vi "CSV2_write portion (SubVI).vi"(5 "format (%.3f)":string="%.3f", 6 "delimiter (\\t)":string="\t", 7 "2D data":dbl[][](array[numeric]) format="%0.2f", 8 "error in (no error)":errorcluster, 9 "transpose? (no:F)":bool, 10 "1D data":dbl[](array[numeric]) format="%0.2f", 11 "File Refnum in":refnum<file>) -> (0 "error out":errorcluster, 3 "File Refnum out":refnum<file>)   [LabVIEW 2012]
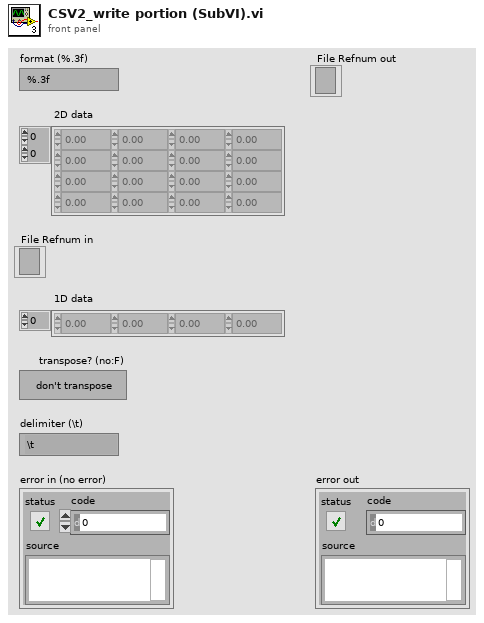
[diagram p1: front panel]
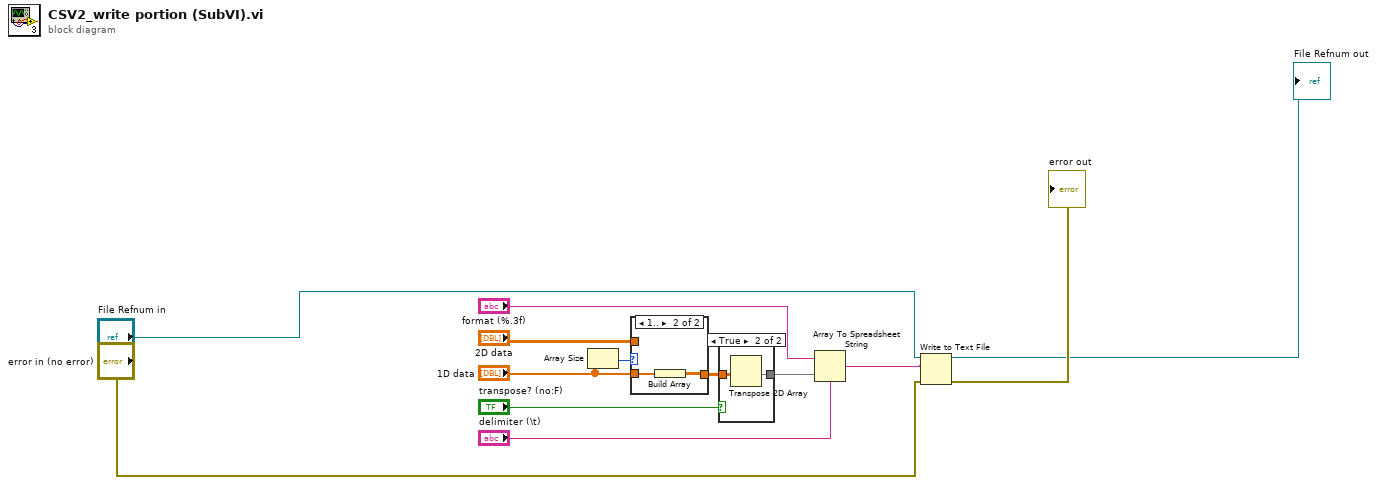
[diagram p0: block diagram]
diagram:
  n1 = Array Size(array="1D data") -> (size(s)=w8:i32)
  n2 = case shown="1.." w8 {
    tunnel: "1D data" -> [_ w16]
    tunnel: [w14 w15] -> w4
    tunnel: "2D data" -> [w14 _]
    frame ..0 {
      # "1D array is empty"
    }
    frame 1.. {
      n3 = Build Array(w16) -> (w15:dbl[][])
    }
  }
  n4 = case shown="True" "transpose? (no:F)" {
    tunnel: [w17 w19] -> w2
    tunnel: w4 -> [w17 w18]
    frame False {
    }
    frame True {
      n5 = Transpose 2D Array(2D array=w18) -> (transposed array=w19:dbl[][])
    }
  }
  n6 = Array To Spreadsheet String(delimiter (Tab)="delimiter (\\t)", array=w2, 3:"format (%.3f)") -> (spreadsheet string=w9:string)
  n7 = Write to Text File(file (use dialog)="File Refnum in", text=w9, error in="error in (no error)") -> (refnum out=→"File Refnum out":refnum<file>, error out=→"error out":errorcluster)  [unwired: 1 in, 1 out]
